vi "FreqMeter_ReadValue.vi"(3 "error in (no error)":errorcluster, 5 "Task ID":u32) -> (0 "error out":errorcluster, 1 "frequency value":dbl, 2 "Task ID":u32)   [LabVIEW 2015]
uses:
  Windows/System32/AdvLvDaq.dll
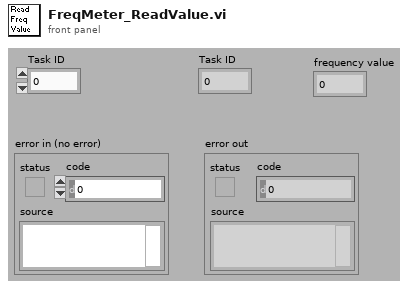
[diagram p1: front panel]
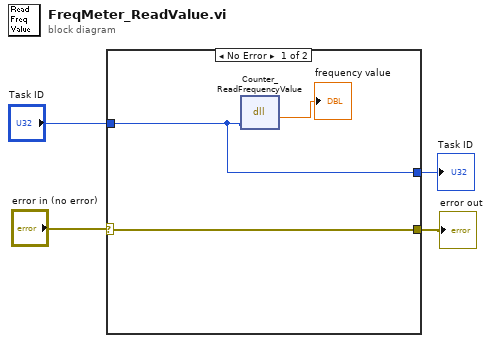
[diagram p0: block diagram]
diagram:
  n1 = case shown="No Error" "error in (no error)" {
    selector: "error in (no error)" -> [w5 w8]
    tunnel: "Task ID" -> [w6 w9]
    tunnel: [w6 w9] -> w2
    tunnel: [w5 w8] -> w1
    frame No Error {
      n2 = dll-call lib="C:/Windows/System32/AdvLvDaq.dll" fn="Counter_ReadFrequencyValue"("taskId"=w6) -> ("return type"=→"frequency value":dbl)  [unwired: 4 in, 2 out]
    }
    frame Error {
    }
  }
  "Task ID" <- w2
  "error out" <- w1
